vi "Call External Interactions.vi"(8 "error in (no error)":errorcluster) -> (0 "error out":errorcluster, 2 "Message":refnum<user-event>, 3 "UUT Result":refnum<user-event>)   [LabVIEW 2019, in "Full User Interface.lvlib"]
uses:
  Full User Interface.lvlib
  Test Unit/UUT Result.ctl
  <vilib>/Test Bench Framework/Test Executive.lvlibp/TestEngine/TestEngine/TestEngine/Typedefs/Report General.ctl
  <vilib>/Test Bench Framework/Test Executive.lvlibp/TestEngine/TestEngine/TestEngine/Test Engine.lvclass
  Test Unit/Test Unit.lvlib
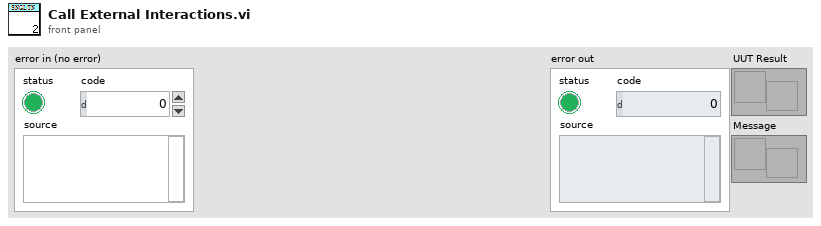
[diagram p1: front panel]
types:
  T1 = typedef "Test Unit.lvlib/UUT Result.ctl" = cluster{"Station":i32, "Socket":i32, "DetailTestResult":string[][], "Report Path":path, "General":T2}
  T2 = typedef "Test Executive.lvlibp/Test Engine.lvlib/Test Engine.lvclass/Report General.ctl" = cluster{"Sequence Path":path, "Serial Number":string, "Test Date Time":timestamp, "UUT Status":string, "Faulty Item":string, "Seconds Executing":dbl}
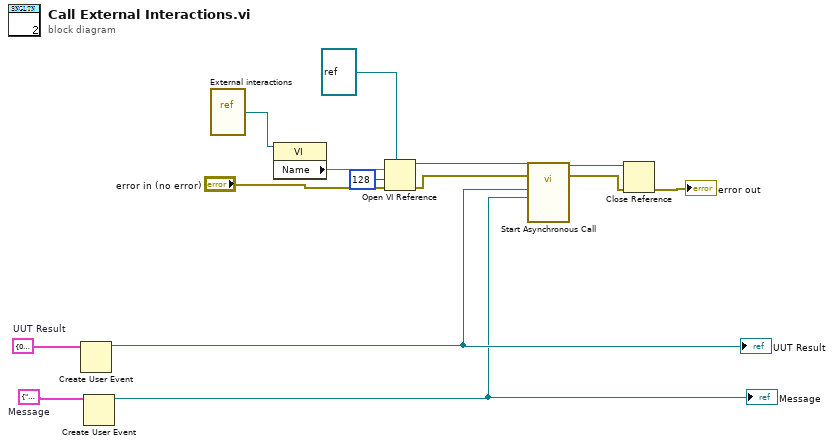
[diagram p0: block diagram]
diagram:
  w13 = cluster{"Msg":string, "Data":variant} {"Msg"="", "Data"=variant}  # Message
  w14 = cluster{"Station":i32, "UUT Result":T1} {"Station"=0, "UUT Result"={"Station"=0, "Socket"=0, "DetailTestResult"=[], "Report Path"=path "", "General"={"Sequence Path"=path "", "Serial Number"="", "Test Date Time"=timestamp(0 s since 1904-01-01), "UUT Status"="", "Faulty Item"="", "Seconds Executing"=0.0}}}  # UUT Result
  n1 = Create User Event(user event datatype=w14) -> (user event=w8:refnum<user-event>)  [unwired: 1 in, 1 out]
  "UUT Result" <- w8
  n2 = Create User Event(user event datatype=w13) -> (user event=w6:refnum<user-event>)  [unwired: 1 in, 1 out]
  "Message" <- w6
  n3 = vi-ref "External interactions.vi"() -> (w12:refnum<vi>)
  n4 = property class="VI"(reference=w12) -> ("Name"=w11:string)  [unwired: 1 in, 2 out]
  n5 = Open VI Reference(type specifier VI Refnum (for type only)=refnum<vi> refnum, vi path=w11, options=128, error in (no error)="error in (no error)") -> (vi reference=w9:refnum<vi>, error out=w7:errorcluster)  [unwired: 2 in]
  n6 = call-by-ref "Start Asynchronous Call"(reference=w9, error in=w7, "Message"=w6, "UUT Result"=w8) -> (reference out=w5:refnum<vi>, error out=w4:errorcluster)  [unwired: 10 in]
  n7 = Close Reference(reference=w5, error in (no error)=w4) -> (error out=→"error out":errorcluster)
